vi "User Updated Status.vi"(8 "error in (no error)":errorcluster, 10 "Status":string, 11 "Chat Window Model in":refnum<class "Chat Window Model.lvclass">) -> (0 "error out":errorcluster, 3 "Chat Window Model out":refnum<class "Chat Window Model.lvclass">)   [LabVIEW 2015, in "Chat Window Model.lvlib" / "Chat Window Model.lvclass"]
uses:
  Chat Window Model.lvclass
  Chat Window Model Messages/Status Updated Msg/Status Updated Msg.lvclass
  <vilib>/ActorFramework/Actor/Actor.lvclass
  Chat Window UI Controller/Chat Window UI Controller Messages/Update VI Title Msg/Update VI Title Msg.lvclass
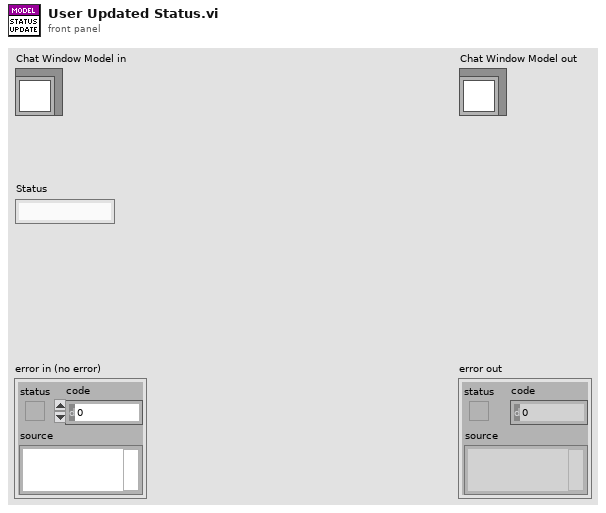
[diagram p1: front panel]
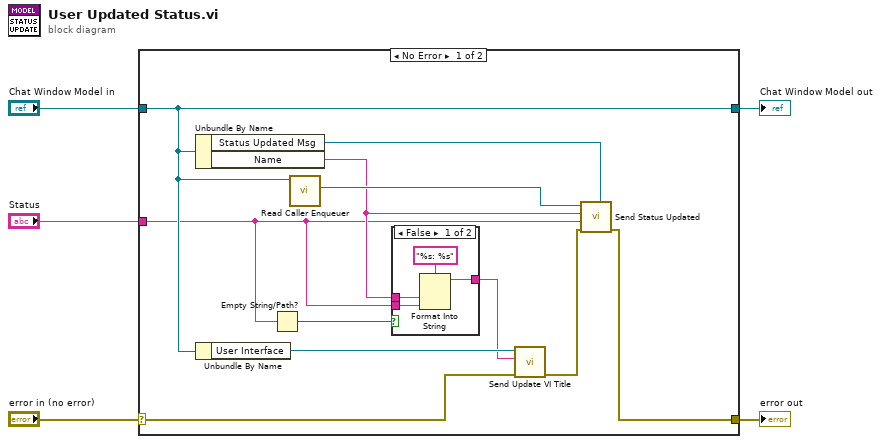
[diagram p0: block diagram]
diagram:
  n1 = case shown="No Error" "error in (no error)" {
    selector: "error in (no error)" -> [w11 w23]
    tunnel: [w14 w23] -> w4
    tunnel: [w13 w22] -> w2
    tunnel: "Chat Window Model in" -> [w13 w22]
    tunnel: "Status" -> [w7 _]
    frame No Error {
      n2 = Unbundle By Name(w13) -> ("Status Updated Msg"=w16:refnum<class "Status Updated Msg.lvclass">, "Name"=w8:string)
      n3 = Unbundle By Name(w13) -> ("User Interface"=w12:refnum<class "Message Enqueuer.lvclass">)
      n4 = Empty String/Path?(string/path=w7) -> (empty?=w6:bool)
      n5 = call <vilib>:"Read Caller Enqueuer.vi"("Actor"=w13) -> ("Caller Enqueuer"=w15:refnum<class "Message Enqueuer.lvclass">)  [unwired: 10 in]
      n6 = case shown="False" w6 {
        tunnel: [w19 w21] -> w9
        tunnel: w8 -> [w18 w21]
        tunnel: w7 -> [w17 _]
        frame False {
          n7 = Format Into String(format string="%s: %s", w18, w17) -> (resulting string=w19:string)  [unwired: 2 in, 1 out]
        }
        frame True {
        }
      }
      n8 = call "Send Update VI Title.vi"("error in (no error)"=w11, "Window Title"=w9, "Message Enqueuer"=w12) -> ("error out"=w10:errorcluster)  [unwired: 7 in, 1 out]
      n9 = call "Send Status Updated.vi"("Message Type"=w16, "error in (no error)"=w10, "Status"=w7, "Name"=w8, "Message Enqueuer"=w15) -> ("error out"=w14:errorcluster)  [unwired: 5 in, 1 out]
    }
    frame Error {
    }
  }
  "error out" <- w4
  "Chat Window Model out" <- w2
